vi "kvCanGetNumberOfChannels.vi"(0 "error in (no error)":errorcluster) -> (1 "Channel Count":i32, 2 "error out":errorcluster)   [LabVIEW 2022 SP3]
doc: "This function returns the number of available CAN channels in the computer. The virtual channels are included in this figure."
uses:
  canlib32.dll
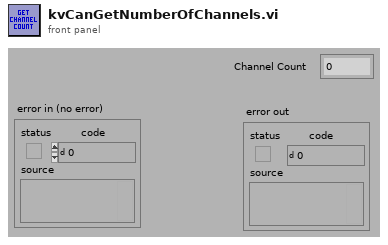
[diagram p1: front panel]
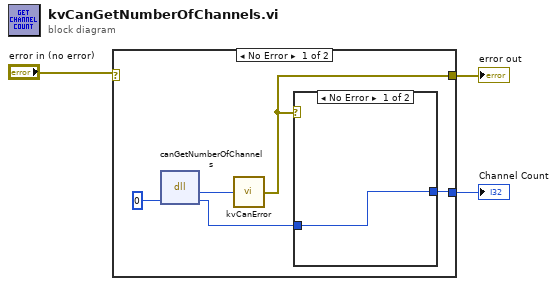
[diagram p0: block diagram]
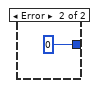
[diagram p2: hidden frame]
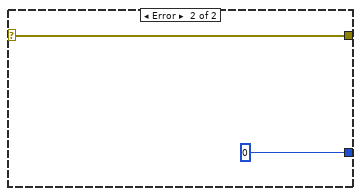
[diagram p3: hidden frame]
diagram:
  n1 = case shown="No Error" "error in (no error)" {
    selector: "error in (no error)" -> [_ w12]
    tunnel: [w6 w12] -> w2
    tunnel: [w5 0] -> w1
    frame No Error {
      n2 = dll-call lib="canlib32.dll" fn="canGetNumberOfChannels"("channelCount"=0) -> (w7:i32, "channelCount"=w4:i32)  [unwired: 3 in, 2 out]
      n3 = call "kvCanError.vi"("error code"=w7) -> ("error out"=w6:errorcluster)
      n4 = case shown="No Error" w6 {
        tunnel: [w9 0] -> w5
        tunnel: w4 -> [w9 _]
        frame No Error {
        }
        frame Error {
        }
      }
    }
    frame Error {
    }
  }
  "error out" <- w2
  "Channel Count" <- w1
